vi "DecimalNumToBinaryString.vi"(11 "十进制 整形":u32) -> (3 "二进制字符串":string)   [LabVIEW 2015]
doc: "本VI把十进制的数值转换为二进制的字符串输出"
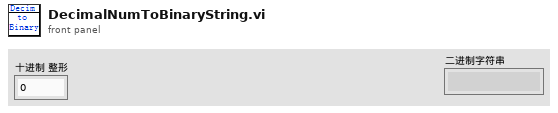
[diagram p1: front panel]
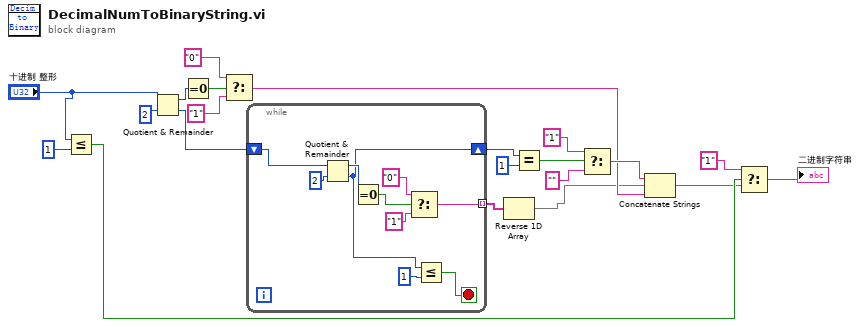
[diagram p0: block diagram]
diagram:
  n1 = Less Or Equal?(x="十进制 整形", y=u32 1) -> (x <= y?=w4:bool)
  n2 = Quotient & Remainder(x="十进制 整形", y=u32 2) -> (x-y*floor(x/y)=w14:u32, floor(x/y)=w20:u32)
  n3 = Equal To 0?(x=w14) -> (x = 0?=w11:bool)
  n4 = Select(t="0", s=w11, f="1") -> (s? t:f=w9:string)
  n5 = while {
    shift-right: [w24] -> w19
    shift-left: w20 -> [w31]
    tunnel: [w25] -> w8 mode=indexing
    stop <- w22 stop-if-true
    n6 = Quotient & Remainder(x=w31, y=u32 2) -> (x-y*floor(x/y)=w29:u32, floor(x/y)=w24:u32)
    n7 = Equal To 0?(x=w29) -> (x = 0?=w28:bool)
    n8 = Select(t="0", s=w28, f="1") -> (s? t:f=w25:string)
    n9 = Less Or Equal?(x=w24, y=u32 1) -> (x <= y?=w22:bool)
  }
  n10 = Reverse 1D Array(array=w8) -> (reversed array=w7:string[])
  n11 = Equal?(x=w19, y=u32 1) -> (x = y?=w17:bool)
  n12 = Select(t="1", s=w17, f="") -> (s? t:f=w10:string)
  n13 = Concatenate Strings(w10, w7, w9) -> (w1:string)
  n14 = Select(t="1", s=w4, f=w1) -> (s? t:f=→"二进制字符串":string)
